vi "Global_SRP_Socket.vi"() -> ()   [LabVIEW 2011]
panel:
  in  "TCP Network Connection Refnum":refnum<k5>
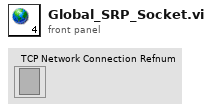
[diagram p1: front panel]
diagram:
